vi "Determine Trigger.vi"(8 "Time Since Last Generation":u32, 9 "Trigger":bool, 10 "Message Parameters":T1={"Generation Type"=enum."Trigger Only", "Period"=1.0, "Include Protection"=FALSE, "Type"=""}, 11 "Enabled":i32) -> (0 "Time Since Last Generation":u32, 1 "Trigger":bool)   [LabVIEW 2013, in "Instrument Addon Engine.lvlib"]
uses:
  Instrument Addon Engine.lvlib
  Shared/Types/Message Parameters.ctl
  Shared/Types/Message Generation Type.ctl
  Shared/Instrument Addon Shared.lvlib
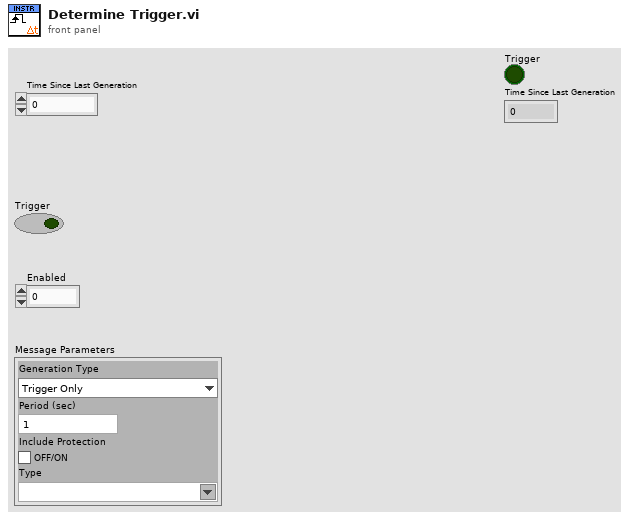
[diagram p1: front panel]
types:
  T1 = typedef "Instrument Addon Shared.lvlib/Message Parameters.ctl" = cluster{"Generation Type":T2, "Period":dbl, "Include Protection":bool, "Type":string}
  T2 = typedef "Instrument Addon Shared.lvlib/Message Generation Type.ctl" = enum16{"Trigger Only", "Periodic & Trigger"}
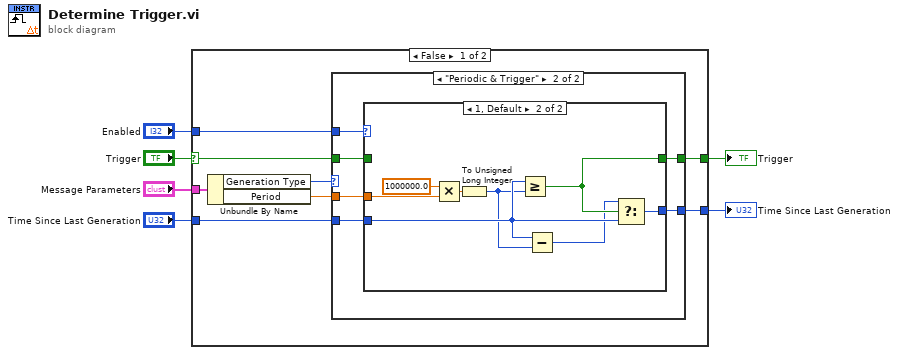
[diagram p0: block diagram]
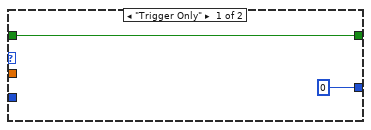
[diagram p2: hidden frame]
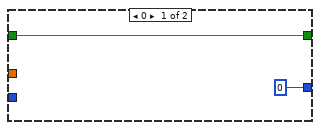
[diagram p3: hidden frame]
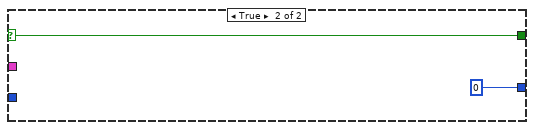
[diagram p4: hidden frame]
diagram:
  n1 = case shown="False" "Trigger" {
    selector: "Trigger" -> [w11 w34]
    tunnel: [w12 w34] -> w2
    tunnel: "Message Parameters" -> [w14 _]
    tunnel: "Enabled" -> [w10 _]
    tunnel: "Time Since Last Generation" -> [w8 _]
    tunnel: [w7 u32 0] -> w1
    frame False {
      n2 = Unbundle By Name(w14) -> ("Generation Type"=w13:T2, "Period"=w9:dbl)
      n3 = case shown="\"Periodic & Trigger\"" w13 {
        tunnel: [w16 w21] -> w12
        tunnel: w11 -> [w16 w20]
        tunnel: w10 -> [_ w22]
        tunnel: w9 -> [_ w19]
        tunnel: w8 -> [_ w18]
        tunnel: [u32 0 w17] -> w7
        frame "Trigger Only" {
        }
        frame "Periodic & Trigger" {
          n4 = case shown="1, Default" w22 {
            tunnel: [w24 w32] -> w21
            tunnel: w20 -> [w24 _]
            tunnel: w19 -> [_ w29]
            tunnel: w18 -> [_ w30]
            tunnel: [u32 0 w31] -> w17
            frame 0 {
            }
            frame 1, Default {
              n5 = Multiply(x=1000000.0, y=w29) -> (x*y=w27:dbl)
              n6 = To Unsigned Long Integer(number=w27) -> (unsigned 32bit integer=w25:u32)
              n7 = Greater Or Equal?(x=w30, y=w25) -> (x >= y?=w32:bool)
              n8 = Subtract(x=w30, y=w25) -> (x-y=w28:u32)
              n9 = Select(t=w28, s=w32, f=w30) -> (s? t:f=w31:u32)
            }
          }
        }
      }
    }
    frame True {
    }
  }
  "Trigger" <- w2
  "Time Since Last Generation" <- w1
